vi "FPS Calculatorv1.vi"() -> (0 "fps":dbl)   [LabVIEW 2013]
doc: "This VI uses a five frame timing window to estimate the frames per second. It is reentrant so that it can be used in multiple locations without interference."
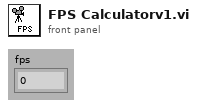
[diagram p1: front panel]
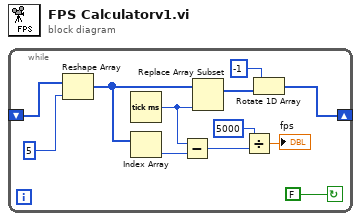
[diagram p0: block diagram]
diagram:
  n1 = while {
    shift-right: [w2] -> _
    shift-left: _ -> [w1]
    stop <- FALSE continue-if-true
    n2 = Reshape Array(w1, 5 ("y")) -> (w4:u32[])
    n3 = Tick Count (ms)() -> (millisecond timer value=w5:u32)
    n4 = Index Array(array=w4) -> (element=w7:u32)  [unwired: 1 in]
    n5 = Subtract(x=w5, y=w7) -> (x-y=w10:u32)
    n6 = Replace Array Subset(array=w4, new element=w5) -> (w3:u32[])  [unwired: 1 in]
    n7 = Divide(x=5000 ("y"), y=w10) -> (x/y=→"fps":dbl)
    n8 = Rotate 1D Array(1:w3, 2:-1 ("y")) -> (0:w2:u32[])
  }
